vi "Read Raw Async Data.vi"(8 "error in (no error)":errorcluster, 10 "Async Message":refnum<class "Async Message.lvclass">, 11 "1553 Component in":refnum<class "1553 Component.lvclass">) -> (0 "error out":errorcluster, 1 "Raw Data":u64[](array[numeric]), 2 "Parameter":string[](array[string]), 3 "1553 Component out":refnum<class "1553 Component.lvclass">)   [LabVIEW 2020, in "BCI-1553 API.lvlib" / "1553 Component.lvclass"]
doc: "Reads the parameters and values associated with an asynchronous message that was sent out on a Bus Controller. Data will be retrieved as raw U64 values.."
uses:
  1553 Component.lvclass
  Frames & Messages/Async Message/Async Message.lvclass
  1553 Component.lvclass/1553 Component.ctl
  Bus Controller/Bus Controller.lvclass
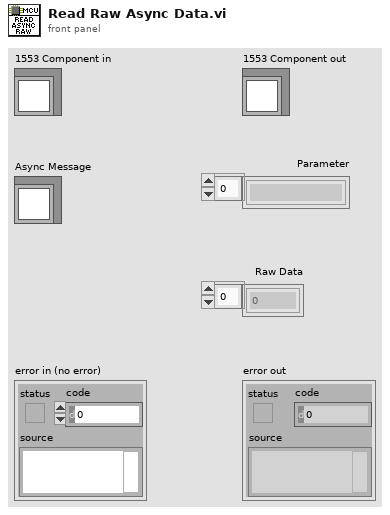
[diagram p1: front panel]
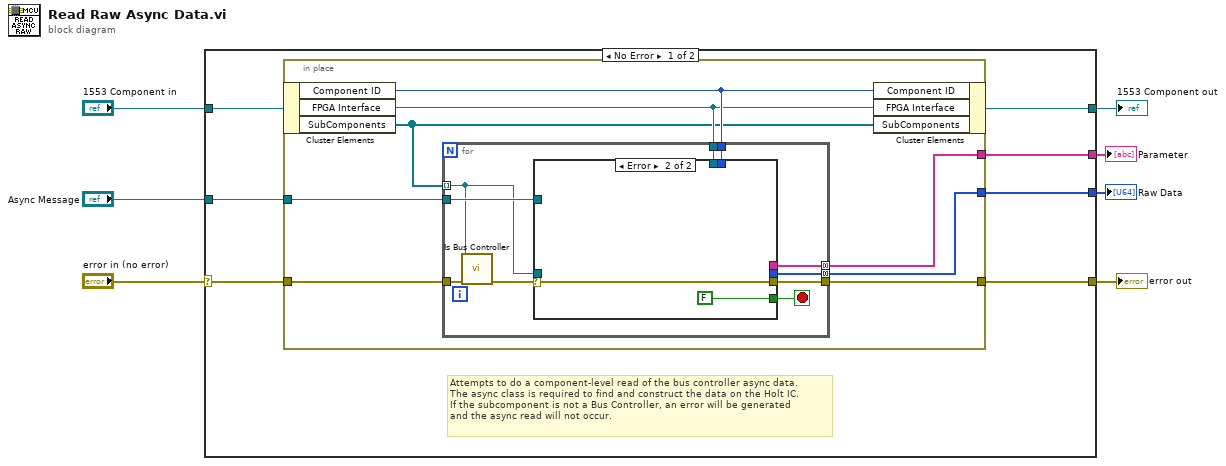
[diagram p0: block diagram]
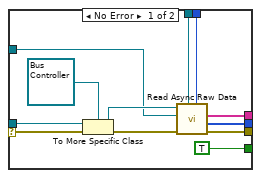
[diagram p2: hidden frame]
diagram:
  n1 = case shown="No Error" "error in (no error)" {
    selector: "error in (no error)" -> [w12 w48]
    tunnel: [w11 w48] -> w6
    tunnel: [w13 w47] -> w4
    tunnel: "1553 Component in" -> [w14 w47]
    tunnel: [w10 _] -> w3
    tunnel: [w9 _] -> w2
    tunnel: "Async Message" -> [w8 _]
    frame No Error {
      # "Attempts to do a component-level read of the bus controller async data.\nThe async class is required to find and construct the data on the Holt IC.\nIf the subcomponent is not a Bus Controller, an error will be generated\nand the async read will not occur."
      n2 = in-place {
        in-place-border: w12 -> [w20]
        in-place-border: [w19] -> w11
        in-place-border: [w18] -> w10
        in-place-border: [w17] -> w9
        in-place-border: w8 -> [w16]
        n3 = in-place-cluster #1(w14) -> ("Component ID"=w22:u8, "FPGA Interface"=w21:refnum<class "FPGA Interface.lvclass">, "SubComponents"=w15:refnum<class "1553 SubComponent.lvclass">[])
        n4 = for {
          tunnel: w15 -> [w23] mode=indexing
          tunnel: w22 -> [w32]
          tunnel: w21 -> [w31]
          tunnel: w20 -> [w27]
          tunnel: [w28] -> w19
          tunnel: [w30] -> w18 mode=concatenating
          tunnel: [w29] -> w17 mode=concatenating
          tunnel: w16 -> [w24]
          stop <- w25 stop-if-true
          n5 = call "Is Bus Controller.vi"("error in (no error)"=w27, "1553 SubComponent"=w23) -> ("error out"=w26:errorcluster)  [unwired: 9 in]
          n6 = case shown="Error" w26 {
            selector: w26 -> [w42 w46]
            tunnel: w32 -> [w34 _]
            tunnel: w31 -> [w35 _]
            tunnel: [w37 _] -> w30
            tunnel: [w36 _] -> w29
            tunnel: [w38 w46] -> w28
            tunnel: w23 -> [w43 _]
            tunnel: [TRUE FALSE] -> w25
            tunnel: w24 -> [w33 _]
            frame No Error {
              n7 = To More Specific Class(target class=refnum<class "Bus Controller.lvclass"> refnum ("SLSC 1553 API.lvlib:Bus Controller.lvclass"), reference=w43, error in=w42) -> (specific class reference=w40:refnum<class "Bus Controller.lvclass">, error out=w39:errorcluster)
              n8 = call-dynamic "Read Async Raw Data.vi"("Component ID"=w34, "FPGA Interface"=w35, "error in (no error)"=w39, "Async Message"=w33, "Bus Controller in"=w40) -> ("error out"=w38:errorcluster, "Parameter Data"=w36:u64[], "Parameters"=w37:string[])  [unwired: 3 in, 1 out]
            }
            frame Error {
            }
          }
        }
        n9 = in-place-cluster #1("Component ID"=w22, "FPGA Interface"=w21, "SubComponents"=w15) -> (w13:refnum<class "1553 Component.lvclass">)
      }
    }
    frame Error {
    }
  }
  "error out" <- w6
  "1553 Component out" <- w4
  "Parameter" <- w3
  "Raw Data" <- w2
